vi "FilterRGBPoly.vi"   [LabVIEW 2024]
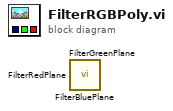
[diagram p0: block diagram]
diagram:
  n1 = call <userlib>:"FilterBluePlane.vi"() -> ()  [unwired: 2 in, 2 out]
  n2 = call <userlib>:"FilterGreenPlane.vi"() -> ()  [unwired: 2 in, 2 out]
  n3 = call <userlib>:"FilterRedPlane.vi"() -> ()  [unwired: 2 in, 2 out]
